vi "Icon_Extract 2D color set.vi"(4 "Width":u32, 6 "Left":i32, 8 "Error":errorcluster, 9 "Height":u32, 10 "Top":i32, 11 "2D Image":T1) -> (0 "Error Out":errorcluster, 3 "2D Image Out":T1)   [LabVIEW 2009]
doc: "Extract 2D Image subset"
uses:
  Controls/Array/Color Box Array_2D Icon Viewer.ctl
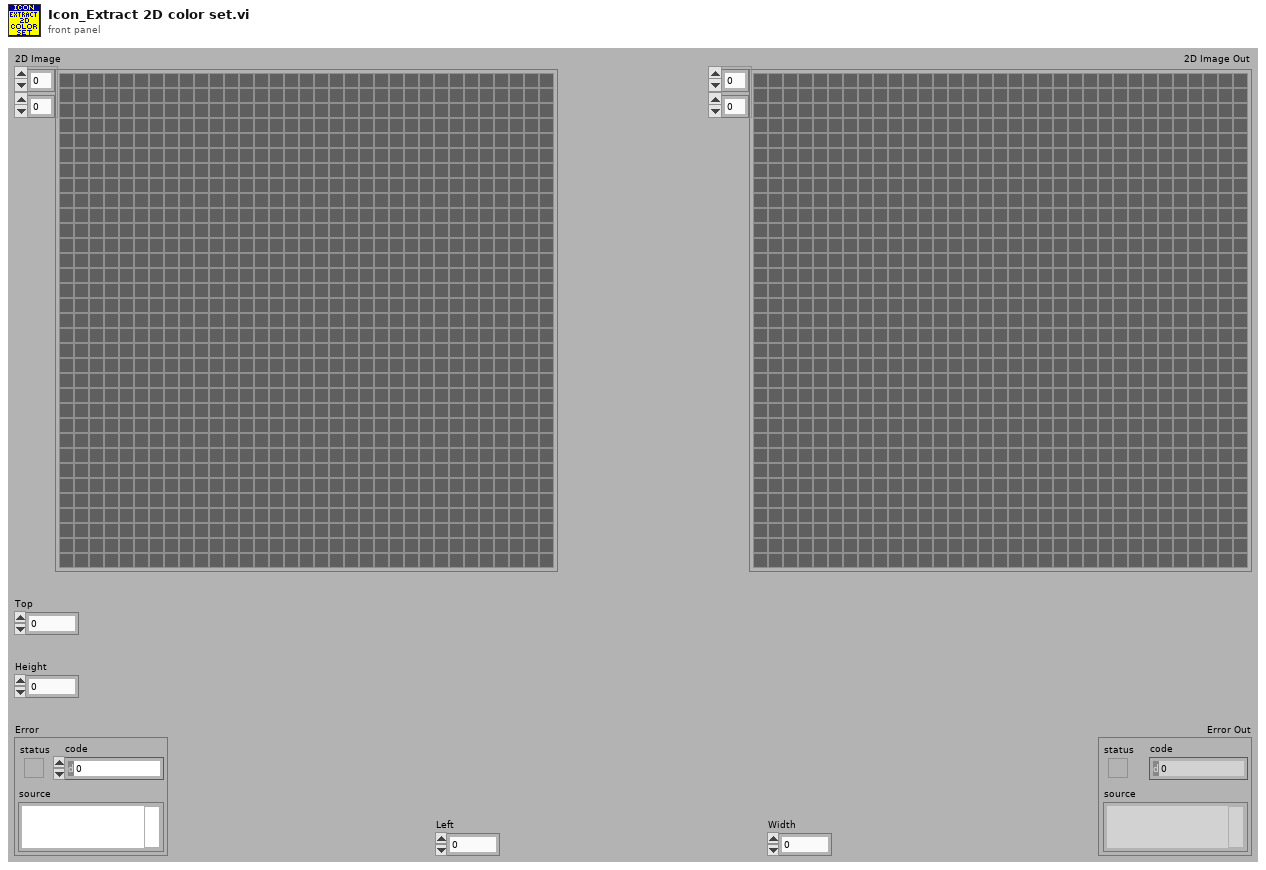
[diagram p1: front panel]
types:
  T1 = typedef "Color Box Array_2D Icon Viewer.ctl" = u32[][]
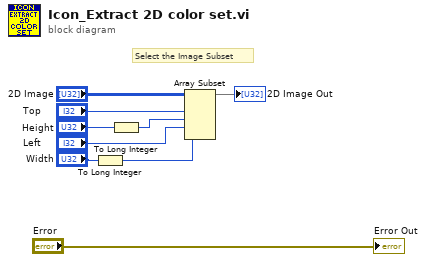
[diagram p0: block diagram]
diagram:
  # "Select the Image Subset"
  n1 = To Long Integer(number="Width") -> (32bit integer=w2:i32)
  n2 = To Long Integer(number="Height") -> (32bit integer=w1:i32)
  n3 = Array Subset(array="2D Image", index (row)="Top", length (row)=w1, index (col)="Left", length (col)=w2) -> (→"2D Image Out":T1)
  "Error Out" <- "Error"
